vi "Save_Mode.vi"(6 "error in (no error)":errorcluster, 9 "Data":T1) -> (0 "error out":errorcluster)   [LabVIEW 2020]
uses:
  <vilib>/Utility/file.llb/Write Delimited Spreadsheet (string).vi
  <vilib>/Utility/file.llb/Write Delimited Spreadsheet (DBL).vi
panel:
  out "cont":i32
  # "SAVE MODE"
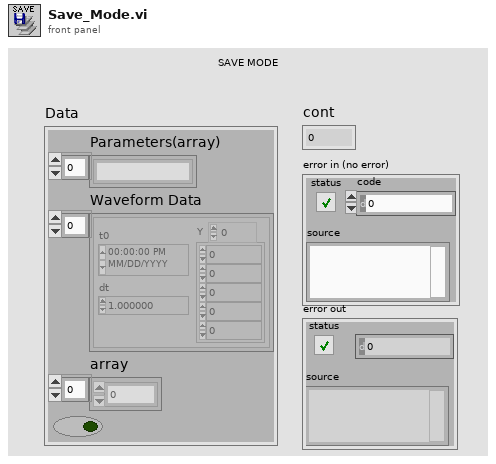
[diagram p1: front panel]
types:
  T1 = cluster{"Parameters(array)":string[], "Waveform Data":waveform(dbl)[], "array":u16[], bool}
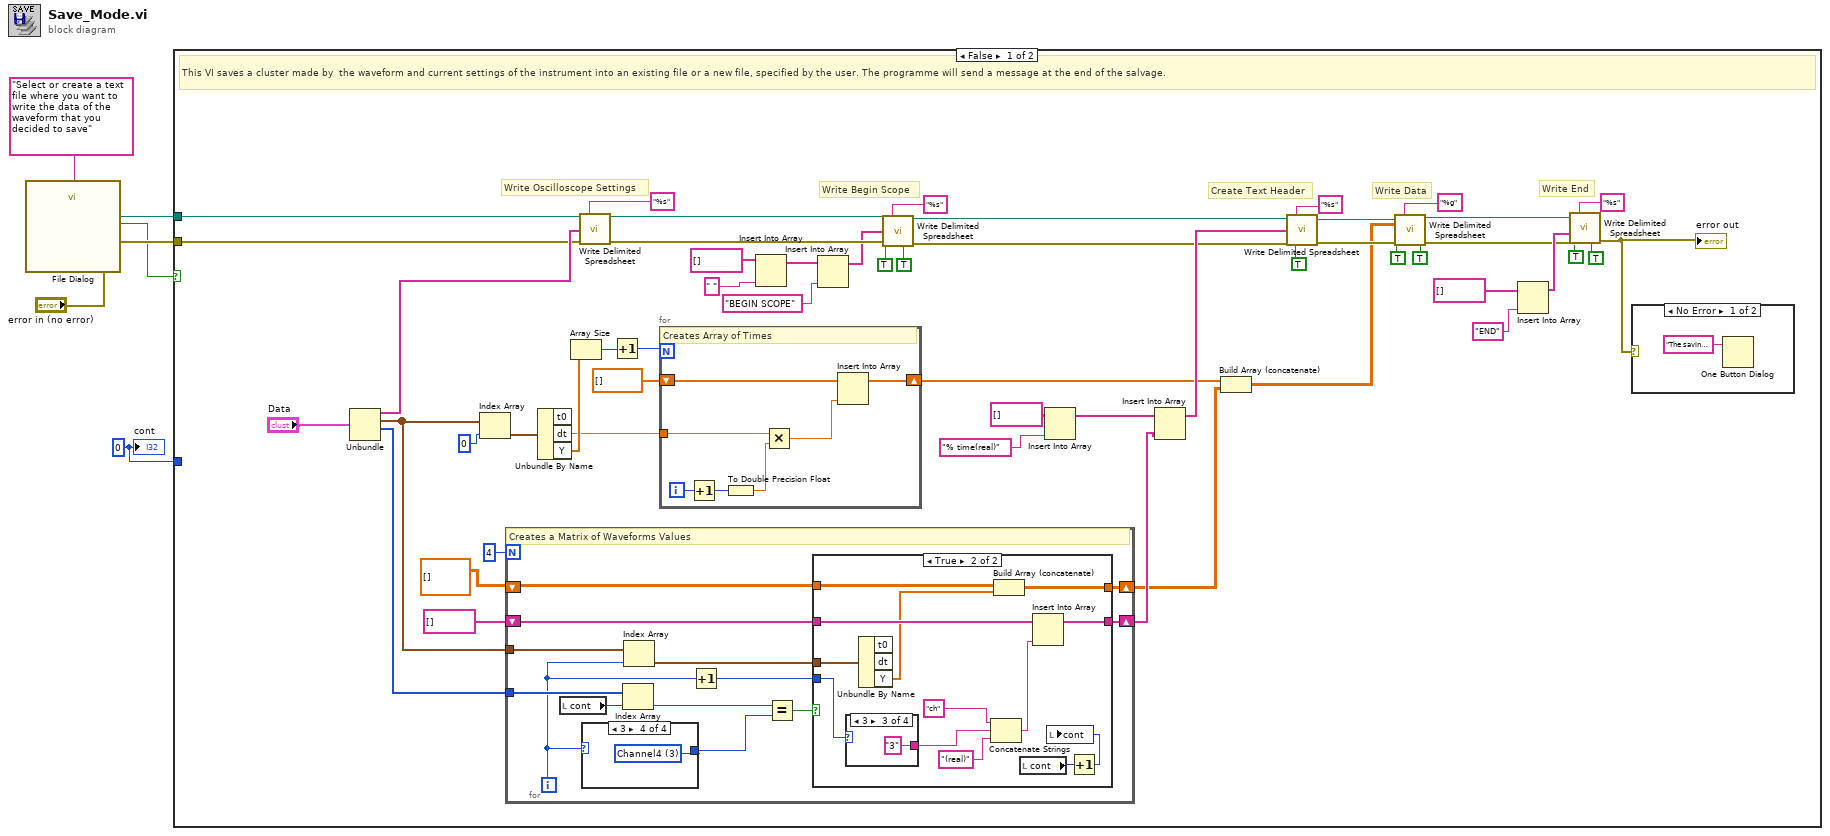
[diagram p0: block diagram]
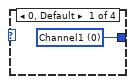
[diagram p2: hidden frame]
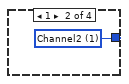
[diagram p3: hidden frame]
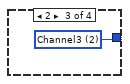
[diagram p4: hidden frame]
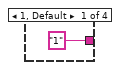
[diagram p6: hidden frame]
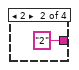
[diagram p7: hidden frame]
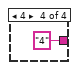
[diagram p8: hidden frame]
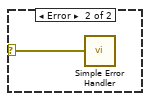
[diagram p9: hidden frame]
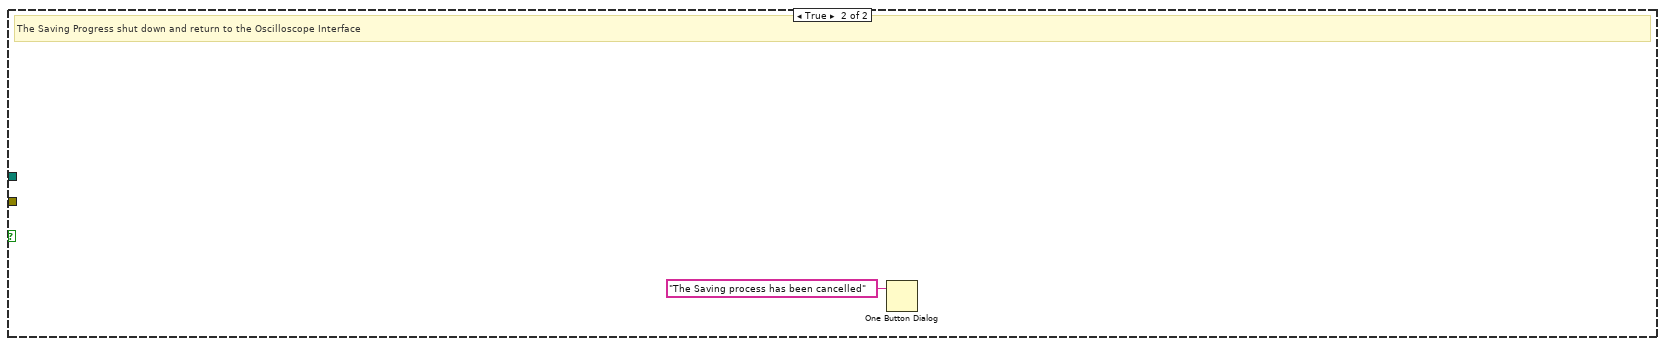
[diagram p10: hidden frame]
diagram:
  w1 = 0 ("cont")
  n1 = call "File Dialog"("prompt"="Select or create a text file where you want to write the data of the waveform that you decided to save" ("prompt (Choose or enter file path)"), "error in"="error in (no error)") -> ("selected path"=w4:path, "cancelled"=w2:bool, "error out"=w3:errorcluster)  [unwired: 10 in, 1 out]
  n2 = case shown="False" w2 {
    tunnel: w4 -> [w50 _]
    tunnel: w3 -> [w49 _]
    tunnel: w1 -> [_ _]
    frame False {
      # "Write End"
      # "Write Begin Scope"
      # "Write Oscilloscope Settings"
      # "Write Data"
      # "Create Text Header"
      # "This VI saves a cluster made by  the waveform and current settings of the instrument into an existing file or a new file, specified by the user. The programme will send a message at the end of the salvage."
      n3 = Unbundle("Data") -> ("Parameters(array)"=w51:string[], "Waveform Data"=w47:waveform(dbl)[], "array"=w53:u16[])  [unwired: 1 out]
      n4 = Index Array(array=w47, index=0) -> (element=w46:waveform(dbl))
      n5 = for {
        N: 4 -> [_]
        tunnel: w47 -> [w79]
        shift-right: [w77] -> w33
        shift-left: dbl[][] [] -> [w68]
        tunnel: w53 -> [w76]
        shift-right: [w71] -> w37
        shift-left: string[] [] -> [w72]
        i -> [w70]
        # "Creates a Matrix of Waveforms Values"
        n6 = local read "cont"() -> (w67:i32)
        n7 = case shown="3" w70 {
          tunnel: [w80 w81 w82 w83] -> w74
          frame 0, Default {
            w80 = u16 0 items=["Channel1", "Channel2", "Channel3", "Channel4", "Math1", "Math2", "Math3", "Math3", "Reference1", "Reference2", "Reference3", "Reference4"] ("Channel (0:Channel1)")
          }
          frame 1 {
            w81 = u16 1 items=["Channel1", "Channel2", "Channel3", "Channel4", "Math1", "Math2", "Math3", "Math3", "Reference1", "Reference2", "Reference3", "Reference4"] ("Channel (0:Channel1)")
          }
          frame 2 {
            w82 = u16 2 items=["Channel1", "Channel2", "Channel3", "Channel4", "Math1", "Math2", "Math3", "Math3", "Reference1", "Reference2", "Reference3", "Reference4"] ("Channel (0:Channel1)")
          }
          frame 3 {
            w83 = u16 3 items=["Channel1", "Channel2", "Channel3", "Channel4", "Math1", "Math2", "Math3", "Math3", "Reference1", "Reference2", "Reference3", "Reference4"] ("Channel (0:Channel1)")
          }
        }
        n8 = Index Array(array=w76, index=w67) -> (element=w75:u16)
        n9 = Index Array(array=w79, index=w70) -> (element=w78:waveform(dbl))
        n10 = Increment(x=w70) -> (x+1=w69:i32)
        n11 = Equal?(x=w75, y=w74) -> (x = y?=w73:bool)
        n12 = case shown="True" w73 {
          tunnel: w78 -> [_ w98]
          tunnel: [w84 w90] -> w77
          tunnel: w72 -> [w85 w92]
          tunnel: [w85 w93] -> w71
          tunnel: w69 -> [_ w96]
          tunnel: w68 -> [w84 w89]
          frame False {
          }
          frame True {
            n13 = case shown="3" w96 {
              tunnel: ["1" "2" "3" "4"] -> w95
              frame 1, Default {
              }
              frame 2 {
              }
              frame 3 {
              }
              frame 4 {
              }
            }
            n14 = Unbundle By Name(w98) -> ("Y"=w88:dbl[])  [unwired: 2 out]
            n15 = Concatenate Strings("ch", w95, "(real)" ("string")) -> (w91:string)
            n16 = Build Array (concatenate)(w89, w88) -> (w90:dbl[][])
            n17 = local read "cont"() -> (w87:i32)
            n18 = Insert Into Array(array=w92, new element=w91) -> (w93:string[])  [unwired: 1 in]
            n19 = Increment(x=w87) -> (x+1=w86:i32)
            n20 = local write "cont"(w86) -> ()
          }
        }
      }
      n21 = Unbundle By Name(w46) -> ("dt"=w44:dbl, "Y"=w45:dbl[])  [unwired: 1 out]
      n22 = Array Size(array=w45) -> (size(s)=w42:i32)
      n23 = call-poly <vilib>:"Write Delimited Spreadsheet.vi"("file path (dialog if empty)"=w50, "format (%s)"="%s" ("format (%.3f)"), "1D data"=w51, "error in (no error)"=w49) -> ("new file path (Not A Path if cancelled)"=w27:path, "error out"=w26:errorcluster)  [unwired: 10 in]
      n24 = Increment(x=w42) -> (x+1=w41:i32)
      n25 = for {
        N: w41 -> [_]
        tunnel: w44 -> [w65]
        shift-right: [w60] -> w35
        shift-left: dbl[] [] ("array") -> [w66]
        i -> [w64]
        # "Creates Array of Times"
        n26 = Increment(x=w64) -> (x+1=w62:i32)
        n27 = To Double Precision Float(number=w62) -> (double precision float=w61:dbl)
        n28 = Multiply(x=w65, y=w61) -> (x*y=w63:dbl)
        n29 = Insert Into Array(array=w66, new element=w63) -> (w60:dbl[])  [unwired: 1 in]
      }
      n30 = Insert Into Array(array=string[] [], new element=" ") -> (w19:string[])  [unwired: 1 in]
      n31 = Insert Into Array(array=w19, new element="BEGIN SCOPE") -> (w15:string[])  [unwired: 1 in]
      n32 = call-poly <vilib>:"Write Delimited Spreadsheet.vi"("file path (dialog if empty)"=w27, "format (%s)"="%s" ("format (%.3f)"), "1D data"=w15, "append to file? (new file:F)"=TRUE, "error in (no error)"=w26, "transpose? (no:F)"=TRUE) -> ("new file path (Not A Path if cancelled)"=w25:path, "error out"=w24:errorcluster)  [unwired: 8 in]
      n33 = Insert Into Array(array=string[] [], new element="% time(real)") -> (w38:string[])  [unwired: 1 in]
      n34 = Insert Into Array(array=w38, new element=w37) -> (w36:string[])  [unwired: 1 in]
      n35 = Build Array (concatenate)(w35, w33) -> (w34:dbl[][])
      n36 = call-poly <vilib>:"Write Delimited Spreadsheet.vi"("file path (dialog if empty)"=w25, "format (%s)"="%s" ("format (%.3f)"), "1D data"=w36, "append to file? (new file:F)"=TRUE, "error in (no error)"=w24) -> ("new file path (Not A Path if cancelled)"=w57:path, "error out"=w54:errorcluster)  [unwired: 9 in]
      n37 = call-poly <vilib>:"Write Delimited Spreadsheet.vi"("file path (dialog if empty)"=w57, "format (%.3f)"="%g", "2D data"=w34, "append to file? (new file:F)"=TRUE, "error in (no error)"=w54, "transpose? (no:F)"=TRUE) -> ("new file path (Not A Path if cancelled)"=w13:path, "error out"=w11:errorcluster)  [unwired: 8 in]
      n38 = Insert Into Array(array=string[] [], new element="END" ("new element/subarray")) -> (w14:string[])  [unwired: 1 in]
      n39 = call-poly <vilib>:"Write Delimited Spreadsheet.vi"("file path (dialog if empty)"=w13, "format (%s)"="%s", "1D data"=w14, "append to file? (new file:F)"=TRUE, "error in (no error)"=w11, "transpose? (no:F)"=TRUE) -> ("error out"=w12:errorcluster)  [unwired: 8 in, 1 out]
      "error out" <- w12
      n40 = case shown="No Error" w12 {
        selector: w12 -> [_ w104]
        frame No Error {
          n41 = One Button Dialog(message="The saving process has been completed") -> ()  [unwired: 1 in, 1 out]
        }
        frame Error {
          n42 = call <vilib>:"Simple Error Handler.vi"("error in (no error)"=w104) -> ()  [unwired: 4 in, 5 out]
        }
      }
    }
    frame True {
      # "The Saving Progress shut down and return to the Oscilloscope Interface"
      n43 = One Button Dialog(message="The Saving process has been cancelled") -> ()  [unwired: 1 in, 1 out]
    }
  }
  "cont" <- w1
